vi "MFCstringFormat.vi"(7 "error in (no error)":errorcluster, 9 "Array":string[](array[string])) -> (0 "error out":errorcluster, 2 "Array out":T1(array[cluster]) {"Setpoint" format="%.2f"; "MassFlow" format="%.2f"})   [LabVIEW 2020]
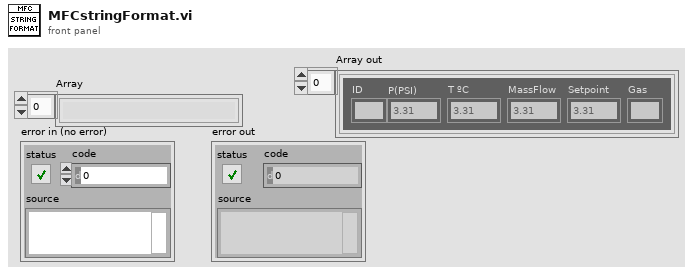
[diagram p1: front panel]
types:
  T1 = cluster{"ID":string, "P(PSI)":dbl, "T ºC":dbl, "MassFlow":dbl, "Setpoint":dbl, "Gas":string}[]
  T2 = cluster{"ID":string, "P(PSI)":dbl, "T ºC":dbl, "MassFlow":dbl, "Setpoint":dbl, "Gas":string}
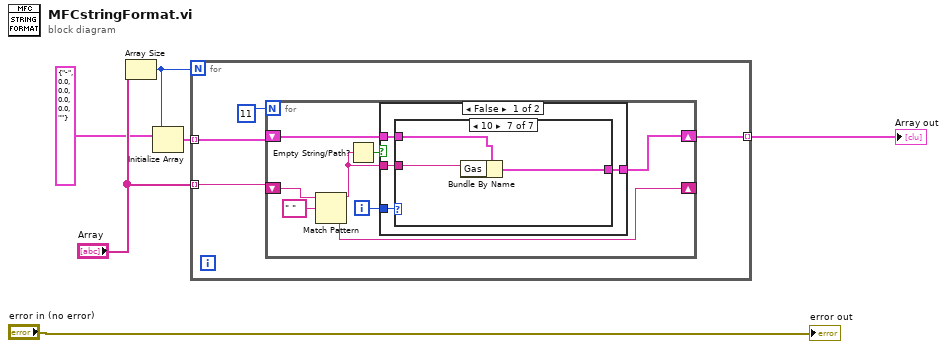
[diagram p0: block diagram]
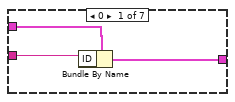
[diagram p2: hidden frame]
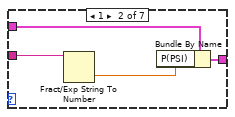
[diagram p3: hidden frame]
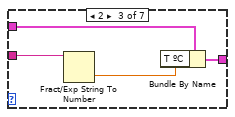
[diagram p4: hidden frame]
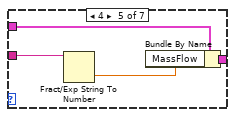
[diagram p6: hidden frame]
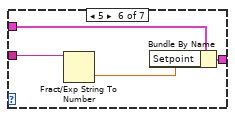
[diagram p7: hidden frame]
diagram:
  n1 = Array Size(array="Array") -> (size(s)=w2:i32)
  n2 = Initialize Array(T2 {"ID"="-", "P(PSI)"=0.0, "T ºC"=0.0, "MassFlow"=0.0, "Setpoint"=0.0, "Gas"=""} ("MFC data"), w2) -> (w1:T1)
  n3 = for {
    N: w2 -> [_]
    tunnel: [w9] -> w6 mode=indexing
    tunnel: "Array" -> [w8] mode=indexing
    tunnel: w1 -> [w7] mode=indexing
    n4 = for {
      N: 11 ("Numeric") -> [_]
      shift-right: [w16] -> _
      shift-left: w8 -> [w18]
      shift-right: [w11] -> w9
      shift-left: w7 -> [w13]
      i -> [w12]
      n5 = Match Pattern(string=w18, regular expression=" ") -> (before substring=w14:string, after substring=w16:string)  [unwired: 1 in, 2 out]
      n6 = Empty String/Path?(string/path=w14) -> (empty?=w15:bool)
      n7 = case shown="False" w15 {
        tunnel: w14 -> [w19 _]
        tunnel: w13 -> [w22 w46]
        tunnel: w12 -> [w21 _]
        tunnel: [w20 w46] -> w11
        frame False {
          n8 = case shown="10" w21 {
            tunnel: w22 -> [w25 w29 w33 w34 w38 w42 w45]
            tunnel: [w24 w28 w32 w34 w37 w41 w44] -> w20
            tunnel: w19 -> [w23 w27 w31 _ w36 w40 w43]
            frame 0 {
              n9 = Bundle By Name(cluster=w25, "ID"=w23) -> (w24:T2)
            }
            frame 1 {
              n10 = Fract/Exp String To Number(string=w27) -> (number=w26:dbl)  [unwired: 3 in, 1 out]
              n11 = Bundle By Name(cluster=w29, "P(PSI)"=w26) -> (w28:T2)
            }
            frame 2 {
              n12 = Fract/Exp String To Number(string=w31) -> (number=w30:dbl)  [unwired: 3 in, 1 out]
              n13 = Bundle By Name(cluster=w33, "T ºC"=w30) -> (w32:T2)
            }
            frame 3, Default {
            }
            frame 4 {
              n14 = Fract/Exp String To Number(string=w36) -> (number=w35:dbl)  [unwired: 3 in, 1 out]
              n15 = Bundle By Name(cluster=w38, "MassFlow"=w35) -> (w37:T2)
            }
            frame 5 {
              n16 = Fract/Exp String To Number(string=w40) -> (number=w39:dbl)  [unwired: 3 in, 1 out]
              n17 = Bundle By Name(cluster=w42, "Setpoint"=w39) -> (w41:T2)
            }
            frame 10 {
              n18 = Bundle By Name(cluster=w45, "Gas"=w43) -> (w44:T2)
            }
          }
        }
        frame True {
        }
      }
    }
  }
  "Array out" <- w6
  "error out" <- "error in (no error)"
